vi "Set_CtrFile.vi"(8 "error in (no error)":errorcluster, 10 "parentTag":T1, 11 "IB_CtrFile in":refnum<class "IB_CtrFile.lvclass">) -> (0 "error out":errorcluster, 3 "IB_CtrFile out":refnum<class "IB_CtrFile.lvclass">)   [LabVIEW 2020, in "IB_CtrFile.lvclass"]
uses:
  <vilib>/AppBuilder/IB_Classes/Source/File/CtrFile/IB_CtrFile.lvclass
  <vilib>/AppBuilder/IB_Classes/Source/File/CtrFile/IB_CtrFile.lvclass/IB_CtrFile.ctl
  <vilib>/AppBuilder/IB_Classes/Source/File/IB_CtrFile.ctl
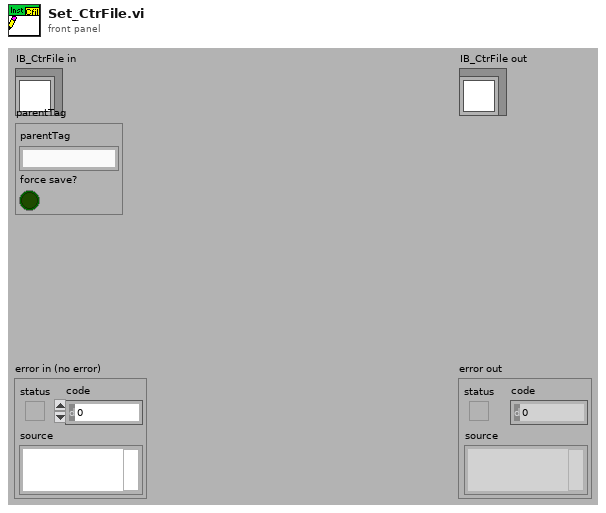
[diagram p1: front panel]
types:
  T1 = typedef "IB_CtrFile.ctl" = cluster{"parentTag":string, "force save?":bool}
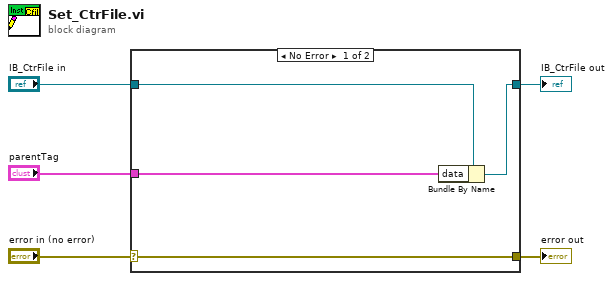
[diagram p0: block diagram]
diagram:
  n1 = case shown="No Error" "error in (no error)" {
    selector: "error in (no error)" -> [w9 w10]
    tunnel: [w9 w10] -> w4
    tunnel: [w7 w11] -> w2
    tunnel: "IB_CtrFile in" -> [w8 w11]
    tunnel: "parentTag" -> [w6 _]
    frame No Error {
      n2 = Bundle By Name(cluster=w8, "data"=w6) -> (w7:refnum<class "IB_CtrFile.lvclass">)
    }
    frame Error {
    }
  }
  "error out" <- w4
  "IB_CtrFile out" <- w2
